vi "JogBase.vi"(4 "connection refnum in":refnum<k5>, 5 "IP Address":string, 6 "error in":errorcluster, 7 "Speed":dbl min=0.0, 8 "Units":enum16{"mm", "µm"}(ring), 9 "Axis":enum16{"Z", "Y", "X"}(ring)) -> (0 "error out":errorcluster, 3 "connection refnum out":refnum<k5>)   [LabVIEW 2023]
doc: "Base function to \"jog\" in a particular axis direction\n\nDo not use this alone. It has no ability to stop the instrument motion.\nYou must use a higher level function with a stop command. JogX, Y, Z are examples of this."
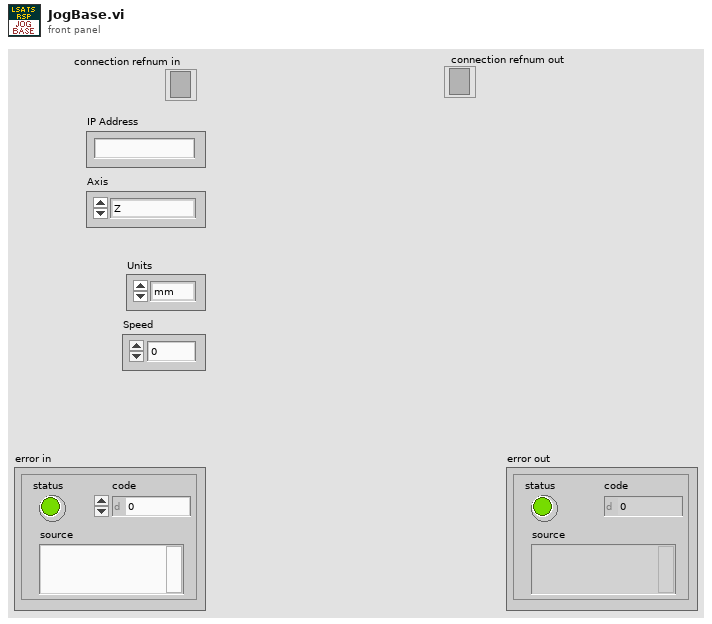
[diagram p1: front panel]
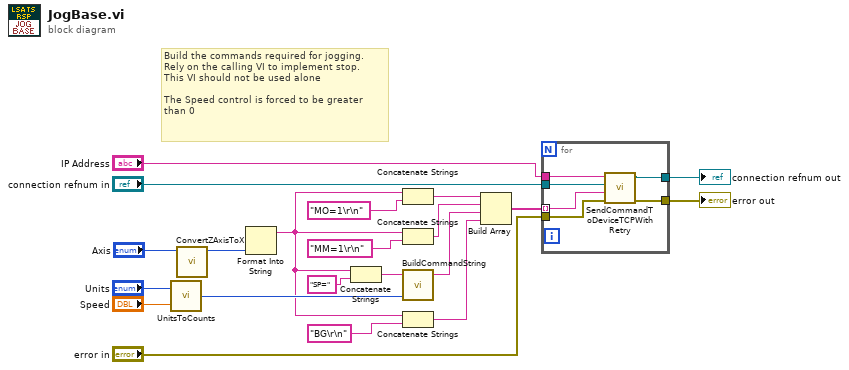
[diagram p0: block diagram]
diagram:
  # "Build the commands required for jogging.\nRely on the calling VI to implement stop.\nThis VI should not be used alone\n\nThe Speed control is forced to be greater than 0"
  n1 = call "UnitsToCounts.vi"("Unit Value"="Speed", "Units"="Units") -> ("Counts"=w18:i32)
  n2 = call "ConvertZAxisToX.vi"("Axis in"="Axis") -> ("Axis out"=w5:enum16{"Z", "Y", "X"})  [unwired: 6 in]
  n3 = Format Into String(w5) -> (resulting string=w8:string)  [unwired: 3 in, 1 out]
  n4 = Concatenate Strings(w8, "SP=") -> (w13:string)
  n5 = Concatenate Strings(w8, "MO=1\r\n") -> (w15:string)
  n6 = Concatenate Strings(w8, "MM=1\r\n") -> (w14:string)
  n7 = call "BuildCommandString.vi"("Numeric Value"=w18, "Command"=w13) -> ("Result"=w11:string)  [unwired: 2 in, 1 out]
  n8 = Concatenate Strings(w8, "BG\r\n") -> (w10:string)
  n9 = Build Array(w15, w14, w11, w10) -> (w20:string[])
  n10 = for {
    tunnel: "IP Address" -> [w26]
    tunnel: [w27] -> w4
    tunnel: w20 -> [w25] mode=indexing
    tunnel: "error in" -> [w24]
    tunnel: "connection refnum in" -> [w23]
    tunnel: [w22] -> w1
    n11 = call "SendCommandToDeviceTCPWithRetry.vi"("error in"=w24, "str command"=w25, "connection refnum in"=w23, "IP address"=w26) -> ("error out"=w27:errorcluster, "connection refnum out"=w22:refnum<k5>)  [unwired: 4 in, 2 out]
  }
  "error out" <- w4
  "connection refnum out" <- w1
